vi "Send Interface Command Event.vi"(8 "error in":errorcluster, 10 "Interface_Command":variant, 11 "Engine in":refnum<class "Engine.lvclass">) -> (0 "error out":errorcluster, 3 "Engine out":refnum<class "Engine.lvclass">)   [LabVIEW 2019, in "Engine.lvlib" / "Engine.lvclass"]
doc: "This routine allows ancestor classes to transmit commands laterally without relying on the actor upsream/downstream relationship (ultimately speeding up data transfer mechanics). The generator and receiver are responsible for verifying the construction of the variant data is correct."
uses:
  Project/Engine.lvclass
  Project/Engine.lvclass/Engine.ctl
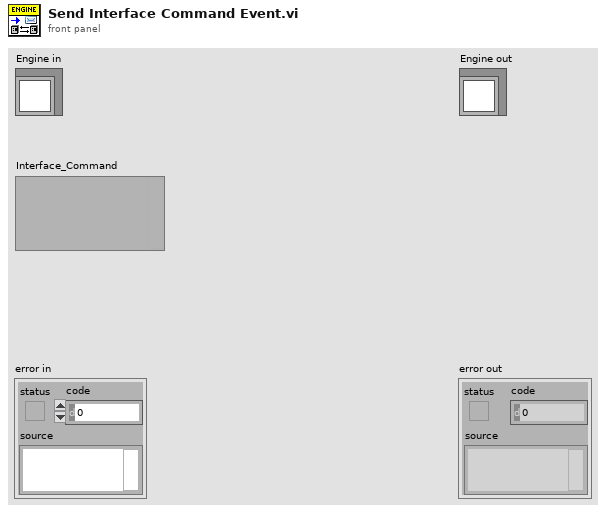
[diagram p1: front panel]
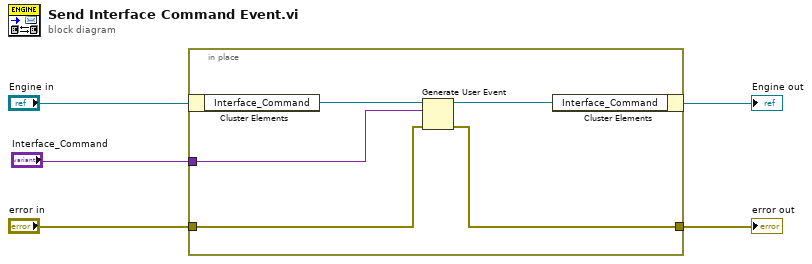
[diagram p0: block diagram]
diagram:
  n1 = in-place {
    in-place-border: "error in" -> [w8]
    in-place-border: [w7] -> w3
    in-place-border: "Interface_Command" -> [w6]
    n2 = in-place-cluster #1("Engine in") -> ("Interface_Command"=w10:refnum<user-event>)
    n3 = Generate User Event(user event=w10, event data cluster=w6, error in=w8) -> (user event out=w9:refnum<user-event>, error out=w7:errorcluster)  [unwired: 1 in]
    n4 = in-place-cluster #1("Interface_Command"=w9) -> (→"Engine out":refnum<class "Engine.lvclass">)
  }
  "error out" <- w3
